vi "VI.GetXCTLS.Libraries.vi"(8 "error in":errorcluster, 10 "All Facade VIs":string[](array[string]), 11 "vi reference":refnum<vi>) -> (0 "error out":errorcluster, 2 "Libraries":refnum<vi>[](array[refnum]), 3 "vi reference out":refnum<vi>)   [LabVIEW 2011]
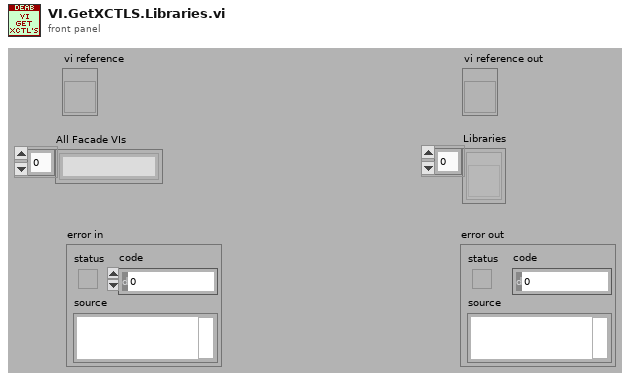
[diagram p1: front panel]
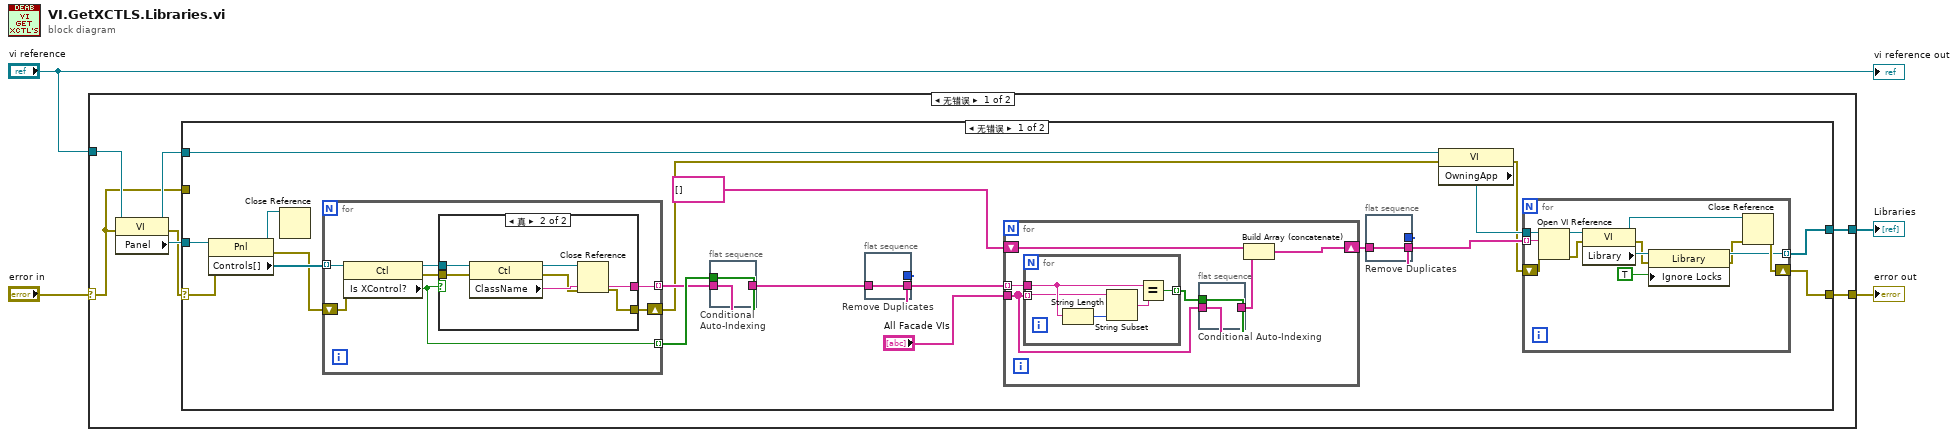
[diagram p0: block diagram]
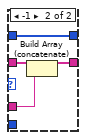
[diagram p2: hidden frame]
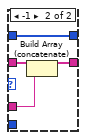
[diagram p3: hidden frame]
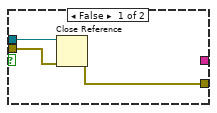
[diagram p4: hidden frame]
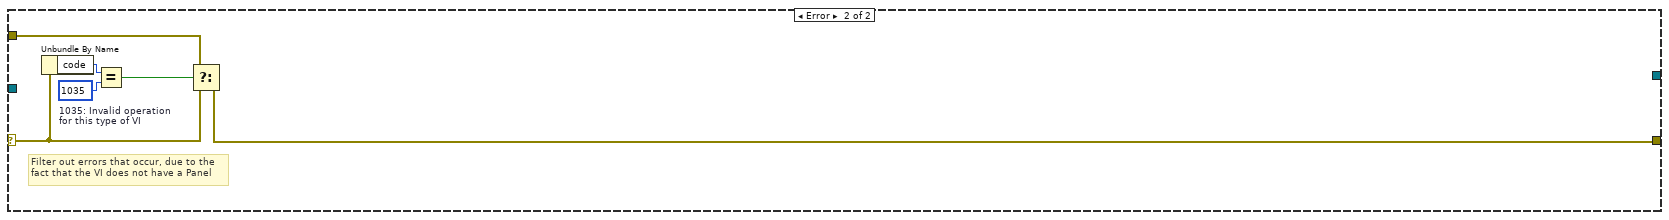
[diagram p5: hidden frame]
diagram:
  n1 = case shown="无错误" "error in" {
    selector: "error in" -> [w5 w144]
    tunnel: "vi reference" -> [w11 _]
    tunnel: [w9 _] -> w4
    tunnel: [w8 w144] -> w3
    frame No Error {
      n2 = property class="VI"(reference=w11, error in=w5) -> (reference out=w7:refnum<vi>, error out=w6:errorcluster, "Panel"=w10:refnum<vi>)
      n3 = case shown="无错误" w6 {
        selector: w6 -> [w12 w139]
        tunnel: w10 -> [w30 _]
        tunnel: [w26 _] -> w9
        tunnel: [w25 w138] -> w8
        tunnel: w7 -> [w17 _]
        tunnel: w5 -> [_ w140]
        frame No Error {
          n4 = property class="Pnl"(reference=w30, error in=w12) -> (reference out=w15:refnum<vi>, error out=w28:errorcluster, "Controls[]"=w29:refnum<vi>[])
          n5 = Close Reference(reference=w15) -> ()  [unwired: 1 in, 1 out]
          n6 = for {
            tunnel: w29 -> [w128] mode=indexing
            tunnel: [w124] -> w23 mode=indexing
            tunnel: [w123] -> w24 mode=indexing
            shift-right: [w122] -> w14
            shift-left: w28 -> [w127]
            n7 = property class="Ctl"(reference=w128, error in=w127) -> (reference out=w126:refnum<vi>, error out=w125:errorcluster, "Is XControl?"=w123:bool)
            n8 = case shown="真" w123 {
              tunnel: w126 -> [w131 w136]
              tunnel: w125 -> [w130 w137]
              tunnel: [_ w135] -> w124
              tunnel: [w129 w132] -> w122
              frame False {
                n9 = Close Reference(reference=w131, error in (no error)=w130) -> (error out=w129:errorcluster)
              }
              frame True {
                n10 = property class="Ctl"(reference=w136, error in=w137) -> (reference out=w134:refnum<vi>, error out=w133:errorcluster, "ClassName"=w135:string)
                n11 = Close Reference(reference=w134, error in (no error)=w133) -> (error out=w132:errorcluster)
              }
            }
          }
          n12 = flat-sequence "Conditional Auto-Indexing" {
            tunnel: w24 -> [w73]
            tunnel: w23 -> [w72]
            tunnel: [w71] -> w22
            frame #0 {
              n13 = Boolean To (0,1)(Boolean=w73) -> (0, 1=w76:i16[])
              n14 = To Unsigned Long Integer(number=w76) -> (unsigned 32bit integer=w77:u32[])
              n15 = Add Array Elements(numeric array=w77) -> (sum=w75:u32)
              n16 = for {
                N: w75 -> [_]
                tunnel: w72 -> [w80]
                tunnel: w73 -> [w84]
                shift-right: [w81] -> _
                shift-left: -1 ("start index (0)") -> [w82]
                tunnel: [w79] -> w71 mode=indexing
                # "index out that element"
                # "Find the next element to keep"
                n17 = Increment(x=w82) -> (x+1=w78:i32)
                n18 = Search 1D Array(1D array=w84, element=TRUE, start index (0)=w78) -> (index of element=w81:i32)
                n19 = Index Array(array=w80, index=w81) -> (element=w79:string)
              }
            }
          }
          n20 = flat-sequence "Remove Duplicates" {
            tunnel: w22 -> [w55]
            tunnel: [w53] -> w21
            tunnel: [w51] -> _
            frame #0 {
              n21 = for {
                tunnel: w55 -> [w61] mode=indexing
                shift-right: [w60] -> w53
                shift-left: string[] [] -> [w59]
                shift-right: [w57] -> w51
                shift-left: i32[] [] -> [w56]
                i -> [w58]
                n22 = Search 1D Array(1D array=w59, element=w61) -> (index of element=w62:i32)  [unwired: 1 in]
                n23 = case shown="Default" w62 {
                  tunnel: w61 -> [_ w70]
                  tunnel: [w66 w68] -> w60
                  tunnel: w59 -> [w66 w69]
                  tunnel: w58 -> [w63 _]
                  tunnel: [w64 w67] -> w57
                  tunnel: w56 -> [w65 w67]
                  frame Default {
                    n24 = Build Array (concatenate)(w65, w63) -> (w64:i32[])
                  }
                  frame -1 {
                    n25 = Build Array (concatenate)(w69, w70) -> (w68:string[])
                  }
                }
              }
            }
          }
          n26 = for {
            tunnel: w21 -> [w102] mode=indexing
            tunnel: "All Facade VIs" -> [w99]
            shift-right: [w100] -> w20
            shift-left: string[] [] -> [w101]
            n27 = for {
              tunnel: w102 -> [w120]
              tunnel: w99 -> [w117] mode=indexing
              tunnel: [w121] -> w98 mode=indexing
              n28 = String Length(string=w120) -> (length=w119:i32)
              n29 = String Subset(string=w117, length (rest)=w119) -> (substring=w118:string)  [unwired: 1 in]
              n30 = Equal?(x=w120, y=w118) -> (x = y?=w121:bool)
            }
            n31 = flat-sequence "Conditional Auto-Indexing" {
              tunnel: w98 -> [w105]
              tunnel: w99 -> [w104]
              tunnel: [w103] -> w97
              frame #0 {
                n32 = Boolean To (0,1)(Boolean=w105) -> (0, 1=w108:i16[])
                n33 = To Unsigned Long Integer(number=w108) -> (unsigned 32bit integer=w109:u32[])
                n34 = Add Array Elements(numeric array=w109) -> (sum=w107:u32)
                n35 = for {
                  N: w107 -> [_]
                  tunnel: w104 -> [w112]
                  tunnel: w105 -> [w116]
                  shift-right: [w113] -> _
                  shift-left: -1 ("start index (0)") -> [w114]
                  tunnel: [w111] -> w103 mode=indexing
                  # "index out that element"
                  # "Find the next element to keep"
                  n36 = Increment(x=w114) -> (x+1=w110:i32)
                  n37 = Search 1D Array(1D array=w116, element=TRUE, start index (0)=w110) -> (index of element=w113:i32)
                  n38 = Index Array(array=w112, index=w113) -> (element=w111:string)
                }
              }
            }
            n39 = Build Array (concatenate)(w101, w97) -> (w100:string[])
          }
          n40 = flat-sequence "Remove Duplicates" {
            tunnel: w20 -> [w35]
            tunnel: [w33] -> w19
            tunnel: [w31] -> _
            frame #0 {
              n41 = for {
                tunnel: w35 -> [w41] mode=indexing
                shift-right: [w40] -> w33
                shift-left: string[] [] -> [w39]
                shift-right: [w37] -> w31
                shift-left: i32[] [] -> [w36]
                i -> [w38]
                n42 = Search 1D Array(1D array=w39, element=w41) -> (index of element=w42:i32)  [unwired: 1 in]
                n43 = case shown="Default" w42 {
                  tunnel: w41 -> [_ w50]
                  tunnel: [w46 w48] -> w40
                  tunnel: w39 -> [w46 w49]
                  tunnel: w38 -> [w43 _]
                  tunnel: [w44 w47] -> w37
                  tunnel: w36 -> [w45 w47]
                  frame Default {
                    n44 = Build Array (concatenate)(w45, w43) -> (w44:i32[])
                  }
                  frame -1 {
                    n45 = Build Array (concatenate)(w49, w50) -> (w48:string[])
                  }
                }
              }
            }
          }
          n46 = property class="VI"(reference=w17, error in=w14) -> (error out=w13:errorcluster, "OwningApp"=w16:refnum<vi>)  [unwired: 1 out]
          n47 = for {
            tunnel: w19 -> [w96] mode=indexing
            tunnel: [w87] -> w26 mode=indexing
            tunnel: w16 -> [w91]
            shift-right: [w92] -> w25
            shift-left: w13 -> [w90]
            n48 = Open VI Reference(application reference (local)=w91, vi path=w96, error in (no error)=w90) -> (vi reference=w95:refnum<vi>, error out=w94:errorcluster)  [unwired: 3 in]
            n49 = property class="VI"(reference=w95, error in=w94) -> (reference out=w93:refnum<vi>, error out=w86:errorcluster, "Library"=w88:refnum<vi>)
            n50 = property class="Library"(reference=w88, error in=w86, "Ignore Locks"=TRUE) -> (reference out=w87:refnum<vi>, error out=w85:errorcluster)
            n51 = Close Reference(reference=w93, error in (no error)=w85) -> (error out=w92:errorcluster)
          }
        }
        frame Error {
          w142 = 1035  # 1035: Invalid operation for this type of VI
          # "Filter out errors that occur, due to the fact that the VI does not have a Panel"
          n52 = Unbundle By Name(w139) -> ("code"=w143:i32)
          n53 = Equal?(x=w143, y=w142) -> (x = y?=w141:bool)
          n54 = Select(t=w140, s=w141, f=w139) -> (s? t:f=w138:errorcluster)
        }
      }
    }
    frame Error {
    }
  }
  "Libraries" <- w4
  "error out" <- w3
  "vi reference out" <- "vi reference"
